vi "Write Interval (ms).vi"(8 "error in (no error)":errorcluster, 10 "Interval (ms)":dbl, 11 "SignalManager in":refnum<class "SignalManager.lvclass">) -> (0 "error out":errorcluster, 3 "SignalManager out":refnum<class "SignalManager.lvclass">)   [LabVIEW 2020, in "SignalManager.lvclass"]
uses:
  SignalManager.lvclass
  SignalManager.lvclass/SignalManager.ctl
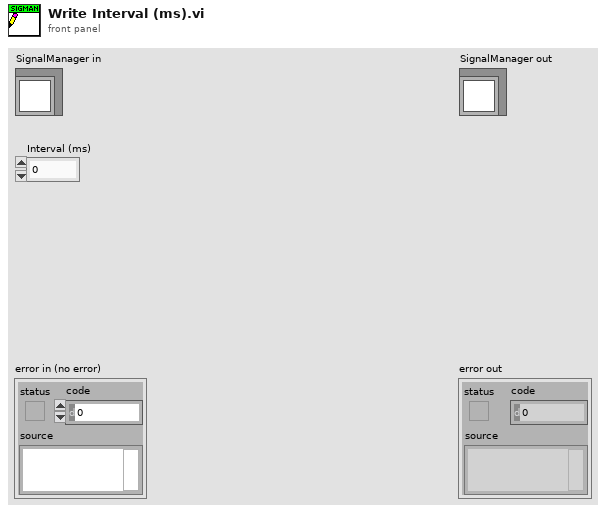
[diagram p1: front panel]
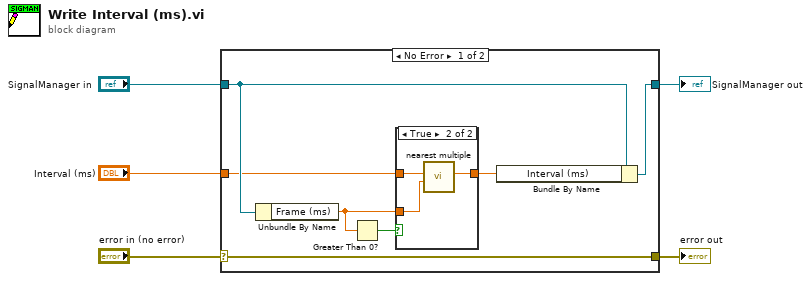
[diagram p0: block diagram]
diagram:
  n1 = case shown="No Error" "error in (no error)" {
    selector: "error in (no error)" -> [w12 w17]
    tunnel: [w12 w17] -> w4
    tunnel: [w11 w18] -> w2
    tunnel: "SignalManager in" -> [w10 w18]
    tunnel: "Interval (ms)" -> [w7 _]
    frame No Error {
      n2 = Unbundle By Name(w10) -> ("Frame (ms)"=w8:dbl)
      n3 = Greater Than 0?(x=w8) -> (x > 0?=w9:bool)
      n4 = case shown="True" w9 {
        tunnel: w8 -> [_ w15]
        tunnel: w7 -> [w13 w16]
        tunnel: [w13 w14] -> w6
        frame False {
        }
        frame True {
          n5 = call "nearest multiple.vi"("y"=w15, "x"=w16) -> ("round(x/y)*y"=w14:dbl)  [unwired: 7 in, 2 out]
        }
      }
      n6 = Bundle By Name(cluster=w10, "Interval (ms)"=w6) -> (w11:refnum<class "SignalManager.lvclass">)
    }
    frame Error {
    }
  }
  "error out" <- w4
  "SignalManager out" <- w2
